vi "UI Max to Normal.vi"(8 "error in (no error)":errorcluster, 10 "Coords":cluster{"Horizontal":i32, "Vertical":i32}, 11 "MainUI in":refnum<class "UI_Top_Customer.lvclass">) -> (0 "error out":errorcluster, 3 "MainUI out":refnum<class "UI_Top_Customer.lvclass">)   [LabVIEW 2021, in "UI_Top_Customer.lvclass"]
uses:
  UI_Top_Customer.lvclass
  UI_Top_Customer.lvclass/UI_Top_Customer.ctl
  <vilib>/Utility/miscctls.llb/LVAllMonitorsDisplayTypeDef.ctl
  <vilib>/Utility/miscctls.llb/LVRectTypeDef.ctl
panel:
  out "Display:Primary Workspace":T1
  out "Display:All Monitors":T2
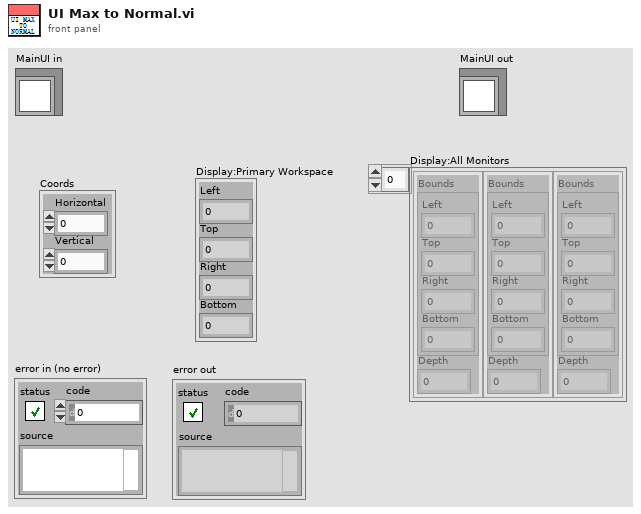
[diagram p1: front panel]
types:
  T1 = typedef "LVRectTypeDef.ctl" = cluster{"Left":i16, "Top":i16, "Right":i16, "Bottom":i16}
  T2 = typedef "LVAllMonitorsDisplayTypeDef.ctl" = cluster{"Bounds":cluster{"Left":i16, "Top":i16, "Right":i16, "Bottom":i16}, "Depth":i16}[]
  T3 = enum32{"Invalid", "Standard", "Closed", "Hidden", "Minimized", "Maximized"}
  T4 = cluster{"Bounds":cluster{"Left":i16, "Top":i16, "Right":i16, "Bottom":i16}, "Depth":i16}
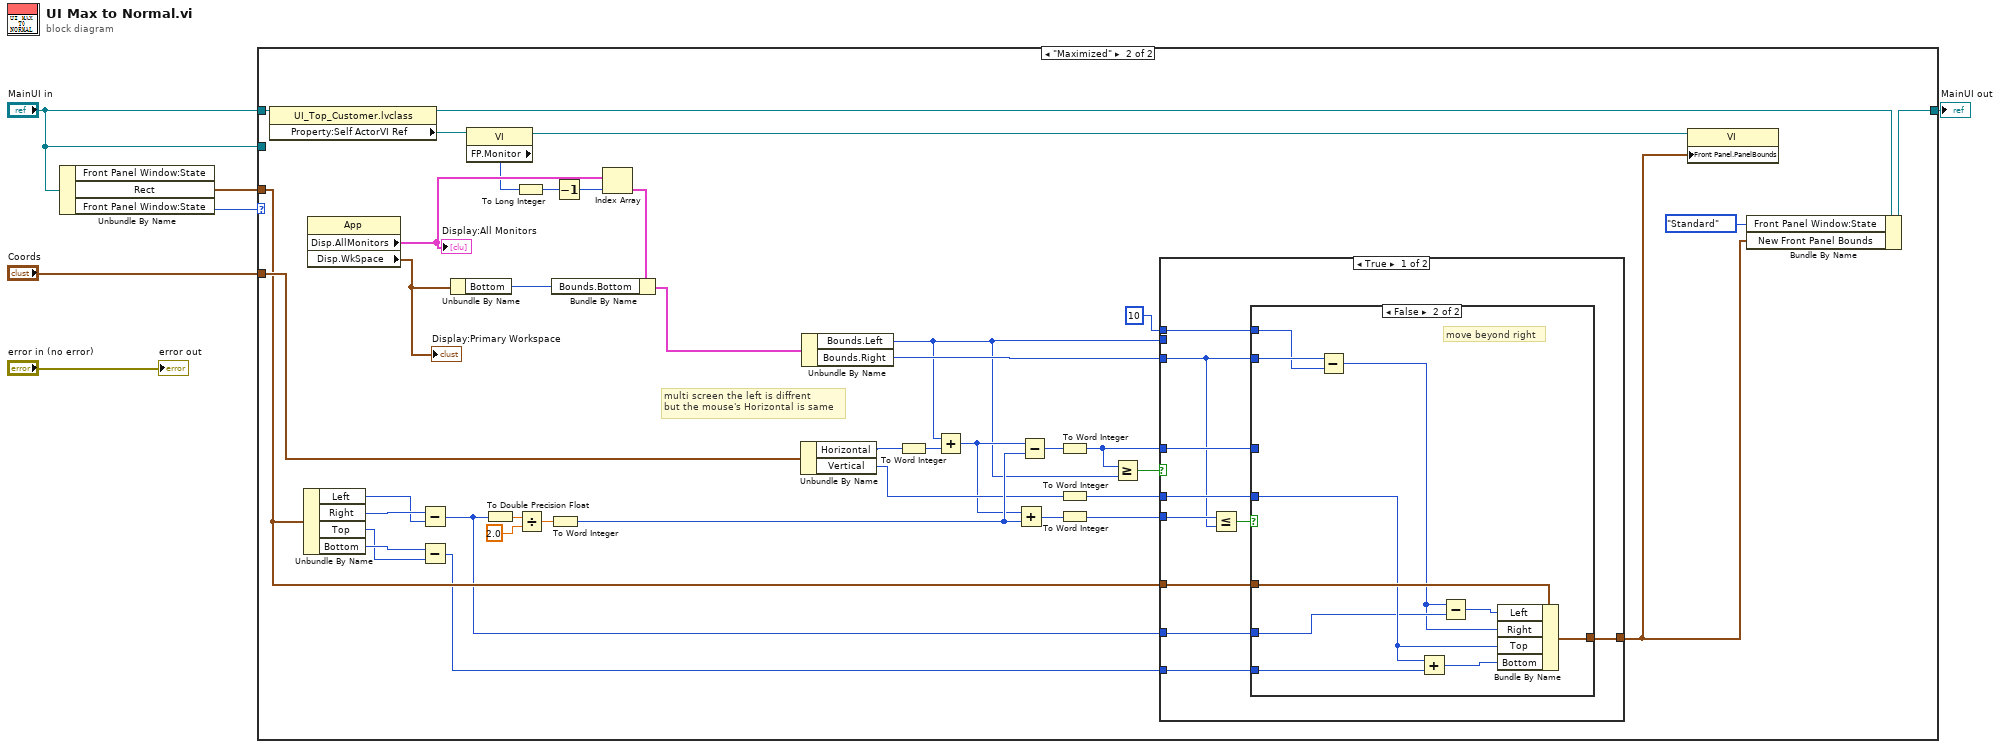
[diagram p0: block diagram]
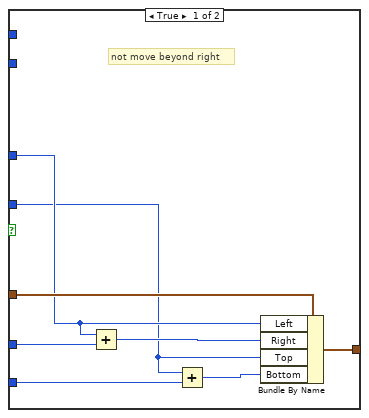
[diagram p3: hidden frame]
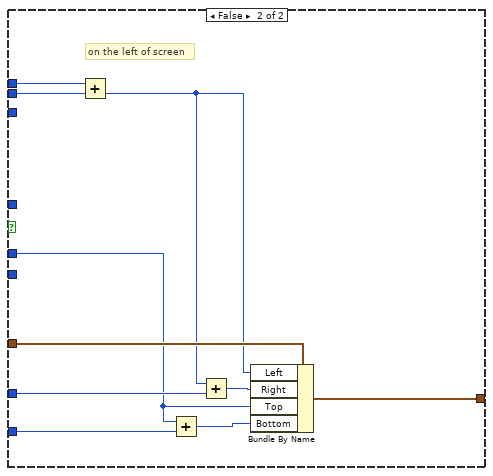
[diagram p4: hidden frame]
diagram:
  n1 = Unbundle By Name("MainUI in") -> ("Rect"=w4:T1, "Front Panel Window:State"=w5:T3)  [unwired: 1 out]
  n2 = case shown="\"Maximized\"" w5 {
    tunnel: w4 -> [_ w26]
    tunnel: "Coords" -> [_ w38]
    tunnel: "MainUI in" -> [_ _]
    tunnel: "MainUI in" -> [w7 w47]
    tunnel: [w7 w9] -> w1
    frame "Invalid", Default {
    }
    frame "Maximized" {
      # "multi screen the left is diffrent\nbut the mouse's Horizontal is same"
      n3 = property class="UI_Top_Customer.lvclass"(reference=w47) -> (reference out=w30:refnum<class "UI_Top_Customer.lvclass">, "Property:Self ActorVI Ref"=w46:refnum<vi>)  [unwired: 1 in, 1 out]
      n4 = Unbundle By Name(w26) -> ("Left"=w36:i16, "Right"=w37:i16, "Top"=w22:i16, "Bottom"=w23:i16)
      n5 = property class="App"() -> ("Disp.AllMonitors"=w45:T2, "Disp.WkSpace"=w40:T1)  [unwired: 2 in, 2 out]
      "Display:All Monitors" <- w45
      "Display:Primary Workspace" <- w40
      n6 = Subtract(x=w37, y=w36) -> (x-y=w24:i16)
      n7 = Subtract(x=w23, y=w22) -> (x-y=w19:i16)
      n8 = Unbundle By Name(w40) -> ("Bottom"=w39:i16)
      n9 = property class="VI"(reference=w46) -> (reference out=w15:refnum<vi>, "FP.Monitor"=w44:u16)  [unwired: 1 in, 1 out]
      n10 = To Double Precision Float(number=w24) -> (double precision float=w35:dbl)
      n11 = To Long Integer(number=w44) -> (32bit integer=w42:i32)
      n12 = Divide(x=w35, y=2.0) -> (x/y=w33:dbl)
      n13 = To Word Integer(number=w33) -> (16bit integer=w31:i16)
      n14 = Decrement(x=w42) -> (x-1=w43:i32)
      n15 = Index Array(array=w45, index=w43) -> (element=w41:T4)
      n16 = Bundle By Name(cluster=w41, "Bounds.Bottom"=w39) -> (w29:T4)
      n17 = Unbundle By Name(w38) -> ("Horizontal"=w32:i32, "Vertical"=w21:i32)
      n18 = Unbundle By Name(w29) -> ("Bounds.Left"=w13:i16, "Bounds.Right"=w18:i16)
      n19 = To Word Integer(number=w32) -> (16bit integer=w12:i16)
      n20 = Add(x=w13, y=w12) -> (x+y=w14:i16)
      n21 = Add(x=w14, y=w31) -> (x+y=w17:i16)
      n22 = Subtract(x=w14, y=w31) -> (x-y=w27:i16)
      n23 = To Word Integer(number=w27) -> (16bit integer=w25:i16)
      n24 = To Word Integer(number=w21) -> (16bit integer=w20:i16)
      n25 = To Word Integer(number=w17) -> (16bit integer=w16:i16)
      n26 = Greater Or Equal?(x=w25, y=w13) -> (x >= y?=w28:bool)
      n27 = case shown="True" w28 {
        tunnel: w25 -> [w55 _]
        tunnel: w26 -> [w57 w85]
        tunnel: w24 -> [w56 w84]
        tunnel: w20 -> [w53 w80]
        tunnel: w19 -> [w54 w82]
        tunnel: w13 -> [_ w79]
        tunnel: w18 -> [w50 _]
        tunnel: w16 -> [w52 _]
        tunnel: [w49 w78] -> w8
        tunnel: i16 10 ("x") -> [w48 w76]
        frame True {
          n28 = Less Or Equal?(x=w52, y=w50) -> (x <= y?=w51:bool)
          n29 = case shown="False" w51 {
            tunnel: w57 -> [w65 w75]
            tunnel: w56 -> [w64 w71]
            tunnel: w55 -> [w62 _]
            tunnel: w54 -> [w61 w74]
            tunnel: w53 -> [w59 w72]
            tunnel: w50 -> [_ w67]
            tunnel: [w58 w69] -> w49
            tunnel: w48 -> [_ w66]
            frame True {
              # "not move beyond right"
              n30 = Add(x=w62, y=w64) -> (x+y=w63:i16)
              n31 = Add(x=w59, y=w61) -> (x+y=w60:i16)
              n32 = Bundle By Name(cluster=w65, "Left"=w62, "Right"=w63, "Top"=w59, "Bottom"=w60) -> (w58:T1)
            }
            frame False {
              # "move beyond right"
              n33 = Subtract(x=w67, y=w66) -> (x-y=w68:i16)
              n34 = Add(x=w72, y=w74) -> (x+y=w73:i16)
              n35 = Subtract(x=w68, y=w71) -> (x-y=w70:i16)
              n36 = Bundle By Name(cluster=w75, "Left"=w70, "Right"=w68, "Top"=w72, "Bottom"=w73) -> (w69:T1)
            }
          }
        }
        frame False {
          # "on the left of screen"
          n37 = Add(x=w76, y=w79) -> (x+y=w77:i16)
          n38 = Add(x=w80, y=w82) -> (x+y=w81:i16)
          n39 = Add(x=w77, y=w84) -> (x+y=w83:i16)
          n40 = Bundle By Name(cluster=w85, "Left"=w77, "Right"=w83, "Top"=w80, "Bottom"=w81) -> (w78:T1)
        }
      }
      n41 = property class="VI"(reference=w15, "Front Panel.PanelBounds"=w8) -> ()  [unwired: 1 in, 2 out]
      n42 = Bundle By Name(cluster=w30, "Front Panel Window:State"=T3."Standard", "New Front Panel Bounds"=w8) -> (w9:refnum<class "UI_Top_Customer.lvclass">)
    }
  }
  "MainUI out" <- w1
  "error out" <- "error in (no error)"
